vi "initialize.vi"(8 "error in (no error)":errorcluster, 11 "Hamamatsu_C9100-13 in":refnum<class "Hamamatsu_C9100-13.lvclass">) -> (0 "error out":errorcluster, 3 "Hamamatsu_C9100-13 out":refnum<class "Hamamatsu_C9100-13.lvclass">)   [LabVIEW 2013, in "Hamamatsu_C9100-13.lvclass"]
uses:
  Hamamatsu_C9100-13.lvclass
  <vilib>/vision/Image Controls.llb/IMAQ Image.ctl
  Hamamatsu_C9100-13.lvclass/Hamamatsu_C9100-13.ctl
  Camera.lvclass
  Globals.vi
panel:
  out "trigger source response":string
  out "trigger mode response":string
  out "Image Buffers Array":T1[](array[typedef])
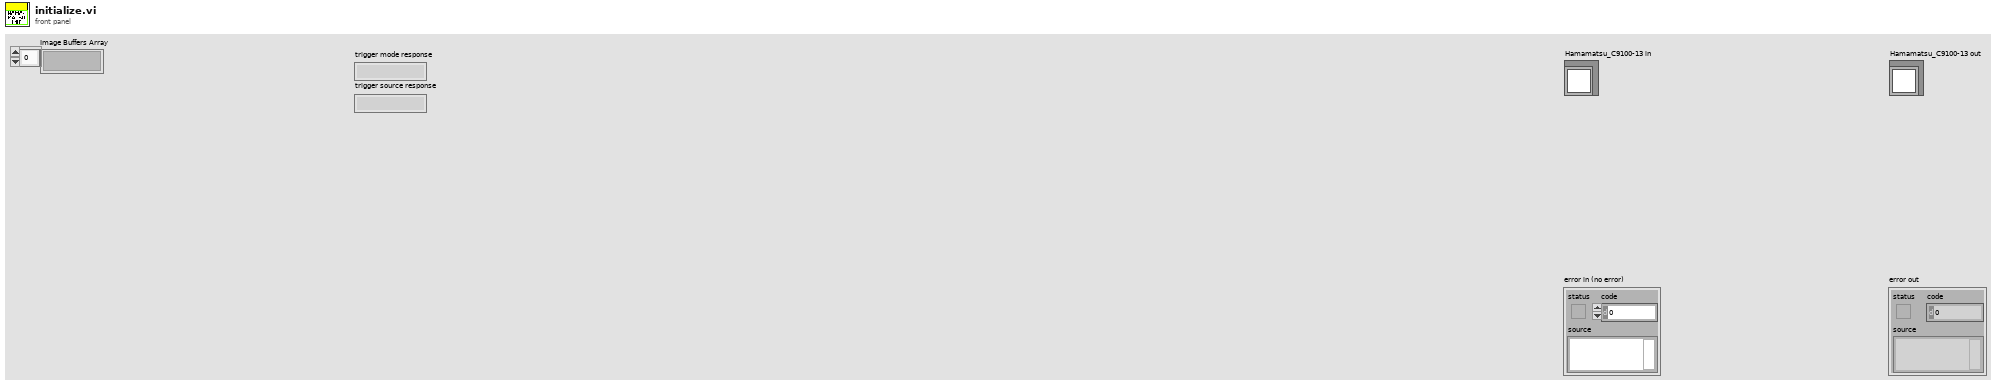
[diagram p1: front panel]
types:
  T1 = typedef "IMAQ Image.ctl" = refnum<image>
  T2 = typedef "Hamamatsu_C9100-13.lvclass/camera_setup.ctl" = cluster{"Analog Gain (0-5)":u8, "Exposure Time":dbl, "EM Gain (0-255)":u8, "Trigger Polarity":string, "External Trigger Mode":string, "Scan Speed":string, "External Trigger Source":string, "Scan Mode":string, "Super Pixel Binning\n(if enabled in Scan Mode)":string, "Camera Sub-array acquisition region\n(if enabled in scan mode)":cluster{"Left":u16, "Top":u16, "Width":u16, "Height":u16}, "Use camera?":bool, "# image buffers":i32, "shots per measurement":i32, "Force images to U16":bool, "Low Light Sensitivity":string, "cooling":string, "fan":string, "Frame Grabber acquisition region":cluster{"Left":i32, "Top":i32, "Right":i32, "Bottom":i32}}
  T3 = cluster{"Left":u16, "Top":u16, "Width":u16, "Height":u16}
  T4 = cluster{"Left":i32, "Top":i32, "Right":i32, "Bottom":i32}
  T5 = typedef "Image Type" = u32
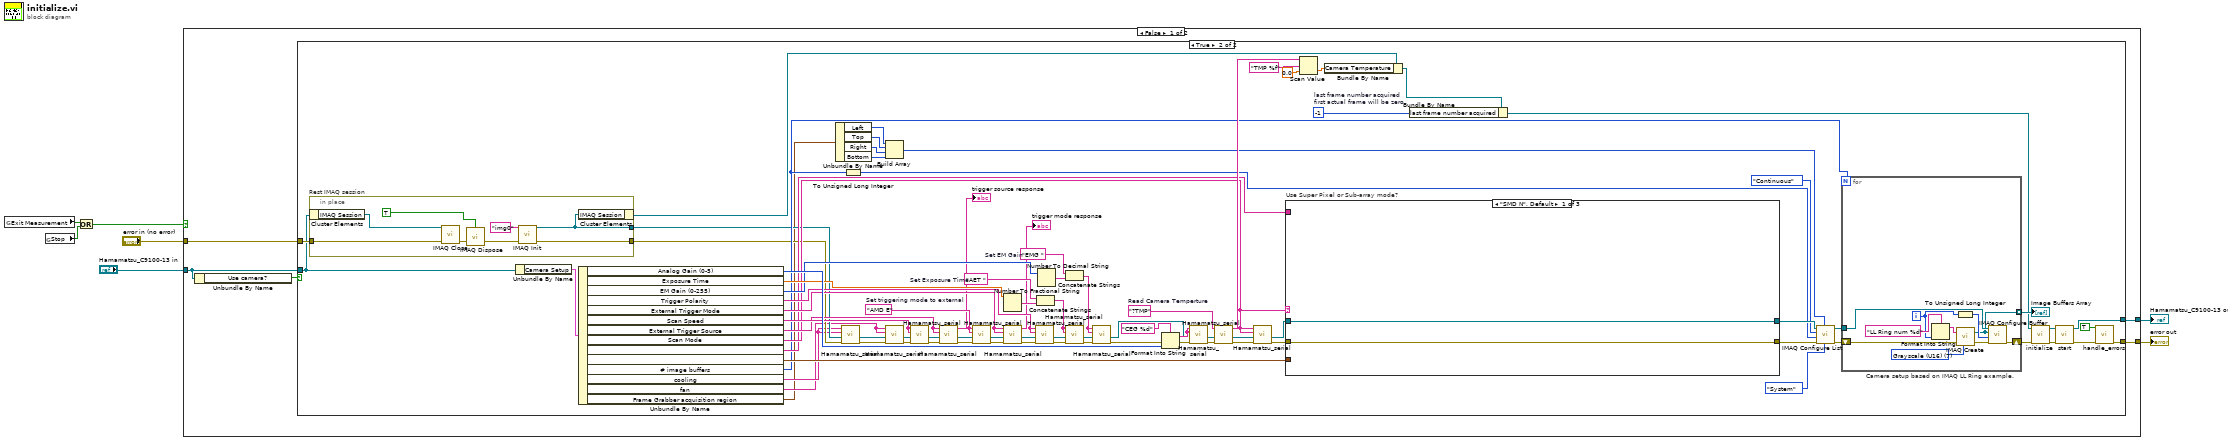
[diagram p0: block diagram]
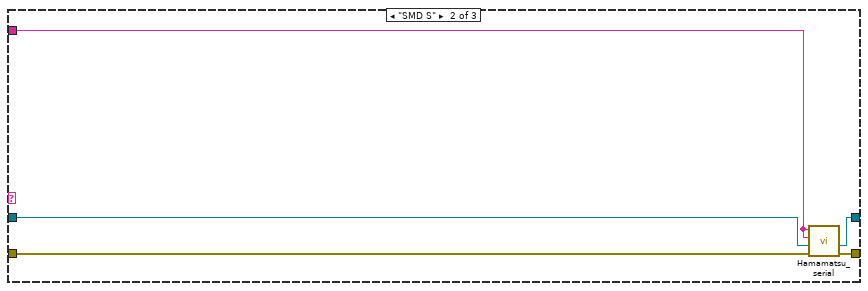
[diagram p3: hidden frame]
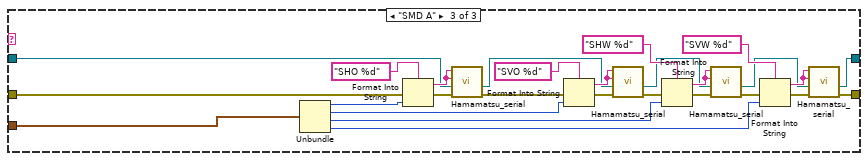
[diagram p4: hidden frame]
diagram:
  n1 = global read "Globals.vi" "Exit Measurement"() -> (w3:bool)
  n2 = global read "Globals.vi" "Stop"() -> (w4:bool)
  n3 = Or(x=w3, y=w4) -> (x .or. y?=w2:bool)
  n4 = case shown="False" w2 {
    tunnel: [w8 w152] -> w7
    tunnel: [w9 w151] -> w6
    tunnel: "Hamamatsu_C9100-13 in" -> [w11 w151]
    tunnel: "error in (no error)" -> [w10 w152]
    frame False {
      n5 = Unbundle By Name(w11) -> ("Use camera?"=w12:bool)
      n6 = case shown="True" w12 {
        tunnel: [w14 w33] -> w8
        tunnel: w10 -> [w14 w17]
        tunnel: w11 -> [w13 w16]
        tunnel: [w13 w30] -> w9
        frame False {
        }
        frame True {
          w22 = -1  # last frame number acquired first actual frame will be zero
          w95 = "EMG "  # Set EM Gain
          w93 = "AET "  # Set Exposure Time
          w88 = "?TMP"  # Read Camera Temperture
          w98 = "AMD E"  # Set triggering mode to external
          n7 = in-place "Rest IMAQ session" {
            in-place-border: [w106] -> w51
            in-place-border: [w99] -> w46
            in-place-border: w17 -> [w102]
            n8 = in-place-cluster #1(w16) -> ("IMAQ Session"=w100:refnum<k11>)
            n9 = call <vilib>:"IMAQ Close.vi"("error in (no error)"=w102, "IMAQ Session In"=w100) -> ("error out"=w101:errorcluster)  [unwired: 9 in]
            n10 = call "IMAQ Dispose"("All Images? (No)"=TRUE, "error in (no error)"=w101) -> ("error out"=w103:errorcluster)  [unwired: 4 in]
            n11 = call <vilib>:"IMAQ Init.vi"("error in (no error)"=w103, "Interface Name"="img0") -> ("error out"=w106:errorcluster, "IMAQ Session Out"=w99:refnum<k11>)  [unwired: 8 in]
            n12 = in-place-cluster #1("IMAQ Session"=w99) -> (w15:refnum<class "Hamamatsu_C9100-13.lvclass">)
          }
          n13 = Unbundle By Name(w16) -> ("Camera Setup"=w37:T2)
          n14 = Unbundle By Name(w37) -> ("Analog Gain (0-5)"=w70:u8, "Exposure Time"=w69:dbl, "EM Gain (0-255)"=w68:u8, "Trigger Polarity"=w67:string, "External Trigger Mode"=w66:string, "Scan Speed"=w65:string, "External Trigger Source"=w64:string, "Scan Mode"=w63:string, "Super Pixel Binning\n(if enabled in Scan Mode)"=w62:string, "Camera Sub-array acquisition region\n(if enabled in scan mode)"=w61:T3, "# image buffers"=w60:i32, "cooling"=w45:string, "fan"=w44:string, "Frame Grabber acquisition region"=w43:T4)
          n15 = Unbundle By Name(w43) -> ("Left"=w42:i32, "Top"=w41:i32, "Right"=w40:i32, "Bottom"=w39:i32)
          n16 = call "Hamamatsu_serial.vi"("error in"=w51, "IMAQ Session In"=w46, "Expected Response"=w45, "Command to send"=w45) -> ("error out"=w50:errorcluster, "IMAQ Session Out"=w47:refnum<k11>)  [unwired: 5 in, 1 out]
          n17 = To Unsigned Long Integer(number=w60) -> (unsigned 32bit integer=w23:u32)
          n18 = Build Array(w42, w41, w40, w39) -> (w38:i32[])
          n19 = call "Hamamatsu_serial.vi"("error in"=w50, "IMAQ Session In"=w47, "Expected Response"=w44, "Command to send"=w44) -> ("error out"=w49:errorcluster, "IMAQ Session Out"=w48:refnum<k11>)  [unwired: 5 in, 1 out]
          n20 = call "Hamamatsu_serial.vi"("error in"=w49, "IMAQ Session In"=w48, "Expected Response"=w65, "Command to send"=w65) -> ("error out"=w79:errorcluster, "IMAQ Session Out"=w80:refnum<k11>)  [unwired: 5 in, 1 out]
          n21 = call "Hamamatsu_serial.vi"("error in"=w79, "IMAQ Session In"=w80, "Expected Response"=w64, "Command to send"=w64) -> ("error out"=w73:errorcluster, "IMAQ Session Out"=w74:refnum<k11>, "Response from Camera"=→"trigger source response":string)  [unwired: 5 in]
          n22 = call "Hamamatsu_serial.vi"("error in"=w73, "IMAQ Session In"=w74, "Expected Response"=w98, "Command to send"=w98) -> ("error out"=w71:errorcluster, "IMAQ Session Out"=w72:refnum<k11>)  [unwired: 5 in, 1 out]
          n23 = Number To Fractional String(number=w69) -> (F-format string=w94:string)  [unwired: 3 in]
          n24 = call "Hamamatsu_serial.vi"("error in"=w71, "IMAQ Session In"=w72, "Expected Response"=w66, "Command to send"=w66) -> ("error out"=w59:errorcluster, "IMAQ Session Out"=w58:refnum<k11>, "Response from Camera"=→"trigger mode response":string)  [unwired: 5 in]
          n25 = call "Hamamatsu_serial.vi"("error in"=w59, "IMAQ Session In"=w58, "Expected Response"=w67, "Command to send"=w67) -> ("error out"=w82:errorcluster, "IMAQ Session Out"=w81:refnum<k11>)  [unwired: 5 in, 1 out]
          n26 = Concatenate Strings(w93, w94) -> (w92:string)
          n27 = Number To Decimal String(number=w68) -> (decimal integer string=w97:string)  [unwired: 1 in]
          n28 = Concatenate Strings(w95, w97) -> (w96:string)
          n29 = call "Hamamatsu_serial.vi"("error in"=w82, "IMAQ Session In"=w81, "Expected Response"=w92, "Command to send"=w92) -> ("error out"=w56:errorcluster, "IMAQ Session Out"=w57:refnum<k11>)  [unwired: 5 in, 1 out]
          n30 = call "Hamamatsu_serial.vi"("error in"=w56, "IMAQ Session In"=w57, "Expected Response"=w96, "Command to send"=w96) -> ("error out"=w84:errorcluster, "IMAQ Session Out"=w83:refnum<k11>)  [unwired: 5 in, 1 out]
          n31 = Format Into String(format string="CEG %d", error in=w84, w70) -> (resulting string=w86:string, error out=w85:errorcluster)  [unwired: 1 in]
          n32 = call "Hamamatsu_serial.vi"("error in"=w85, "IMAQ Session In"=w83, "Expected Response"=w86, "Command to send"=w86) -> ("error out"=w55:errorcluster, "IMAQ Session Out"=w54:refnum<k11>)  [unwired: 5 in, 1 out]
          n33 = call "Hamamatsu_serial.vi"("error in"=w55, "IMAQ Session In"=w54, "Command to send"=w88) -> ("error out"=w78:errorcluster, "IMAQ Session Out"=w76:refnum<k11>, "Response from Camera"=w90:string)  [unwired: 6 in]
          n34 = call "Hamamatsu_serial.vi"("error in"=w78, "IMAQ Session In"=w76, "Expected Response"=w63, "Command to send"=w63) -> ("error out"=w77:errorcluster, "IMAQ Session Out"=w75:refnum<k11>)  [unwired: 5 in, 1 out]
          n35 = case "Use Super Pixel or Sub-array mode?" shown="\"SMD N\", Default" w63 {
            tunnel: w77 -> [w118 w123 w130]
            tunnel: [w118 w122 w131] -> w53
            tunnel: [w117 w119 w132] -> w52
            tunnel: w75 -> [w117 w120 w129]
            tunnel: w62 -> [_ w121 _]
            tunnel: w61 -> [_ _ w128]
            frame "SMD N", Default {
            }
            frame "SMD S" {
              n36 = call "Hamamatsu_serial.vi"("error in"=w123, "IMAQ Session In"=w120, "Expected Response"=w121, "Command to send"=w121) -> ("error out"=w122:errorcluster, "IMAQ Session Out"=w119:refnum<k11>)  [unwired: 5 in, 1 out]
            }
            frame "SMD A" {
              n37 = Unbundle(w128) -> ("Left"=w127:u16, "Top"=w126:u16, "Width"=w125:u16, "Height"=w124:u16)
              n38 = Format Into String(format string="SHO %d", error in=w130, w127) -> (resulting string=w147:string, error out=w137:errorcluster)  [unwired: 1 in]
              n39 = call "Hamamatsu_serial.vi"("error in"=w137, "IMAQ Session In"=w129, "Expected Response"=w147, "Command to send"=w147) -> ("error out"=w138:errorcluster, "IMAQ Session Out"=w135:refnum<k11>)  [unwired: 5 in, 1 out]
              n40 = Format Into String(format string="SVO %d", error in=w138, w126) -> (resulting string=w148:string, error out=w139:errorcluster)  [unwired: 1 in]
              n41 = call "Hamamatsu_serial.vi"("error in"=w139, "IMAQ Session In"=w135, "Expected Response"=w148, "Command to send"=w148) -> ("error out"=w140:errorcluster, "IMAQ Session Out"=w134:refnum<k11>)  [unwired: 5 in, 1 out]
              n42 = Format Into String(format string="SHW %d", error in=w140, w125) -> (resulting string=w149:string, error out=w141:errorcluster)  [unwired: 1 in]
              n43 = call "Hamamatsu_serial.vi"("error in"=w141, "IMAQ Session In"=w134, "Expected Response"=w149, "Command to send"=w149) -> ("error out"=w142:errorcluster, "IMAQ Session Out"=w133:refnum<k11>)  [unwired: 5 in, 1 out]
              n44 = Format Into String(format string="SVW %d", error in=w142, w124) -> (resulting string=w150:string, error out=w143:errorcluster)  [unwired: 1 in]
              n45 = call "Hamamatsu_serial.vi"("error in"=w143, "IMAQ Session In"=w133, "Expected Response"=w150, "Command to send"=w150) -> ("error out"=w131:errorcluster, "IMAQ Session Out"=w132:refnum<k11>)  [unwired: 5 in, 1 out]
            }
          }
          n46 = Scan Value(string=w90, format string="TMP %f", default (0 dbl)=0.0 ("value (0)")) -> (value=w35:dbl)  [unwired: 1 out]
          n47 = Bundle By Name(cluster=w15, "Camera Temperature"=w35) -> (w36:refnum<class "Hamamatsu_C9100-13.lvclass">)
          n48 = Bundle By Name(cluster=w36, "last frame number acquired"=w22) -> (w21:refnum<class "Hamamatsu_C9100-13.lvclass">)
          n49 = call <vilib>:"IMAQ Configure List.vi"("Memory Location"=enum16{"System", "Onboard"}."System", "Region of interest"=w38, "error in (no error)"=w53, "Number of buffers"=w23, "Continuous?"=enum16{"One-Shot", "Continuous"}."Continuous", "IMAQ Session In"=w52) -> ("error out"=w25:errorcluster, "IMAQ Session Out"=w26:refnum<k11>)  [unwired: 4 in]
          n50 = for "Camera setup based on IMAQ LL Ring example." {
            N: w60 -> [_]
            tunnel: w26 -> [w115]
            shift-right: [w112] -> w20
            shift-left: w25 -> [w116]
            tunnel: [w107] -> w27 mode=indexing
            i -> [w110]
            w111 = T5 7 items=["Grayscale (U8)", "Grayscale (I16)", "Grayscale (SGL)", "Complex (CSG)", "RGB (U32)", "HSL (U32)", "RGB (U64)", "Grayscale (U16)"] ("Image Type")
            n51 = Format Into String(format string="LL Ring num %d", w110) -> (resulting string=w114:string)  [unwired: 2 in, 1 out]
            n52 = To Unsigned Long Integer(number=w110) -> (unsigned 32bit integer=w109:u32)
            n53 = call "IMAQ Create"("Image Name"=w114, "Image Type"=w111, "error in (no error)"=w116) -> ("New Image"=w107:T1, "error out"=w108:errorcluster)  [unwired: 2 in]
            n54 = call <vilib>:"IMAQ Configure Buffer.vi"("error in (no error)"=w108, "Buffer Number"=w109, "Image In"=w107, "IMAQ Session In"=w115) -> ("error out"=w112:errorcluster)  [unwired: 6 in, 1 out]
          }
          "Image Buffers Array" <- w27
          n55 = call-parent "initialize.vi"("error in (no error)"=w20, "Camera in"=w21) -> ("error out"=w19:errorcluster, "Camera out"=w18:refnum<class "Hamamatsu_C9100-13.lvclass">)  [unwired: 8 in]
          n56 = call-dynamic "start.vi"("error in (no error)"=w19, "Hamamatsu_C9100-13 in"=w18) -> ("error out"=w29:errorcluster, "Hamamatsu_C9100-13 out"=w30:refnum<class "Hamamatsu_C9100-13.lvclass">)  [unwired: 8 in]
          n57 = call "handle_errors.vi"("Exit Operation"=TRUE, "error in (no error)"=w29) -> ("error out"=w33:errorcluster)  [unwired: 13 in]
        }
      }
    }
    frame True {
    }
  }
  "error out" <- w7
  "Hamamatsu_C9100-13 out" <- w6
